vi "未命名 2.vi"() -> ()   [LabVIEW 2010]
panel:
  out "bStop":bool
  out "bRece":bool
  out "bSend":bool
  out "tmp":string
  out "第几个":i32
  out "第几组":i32
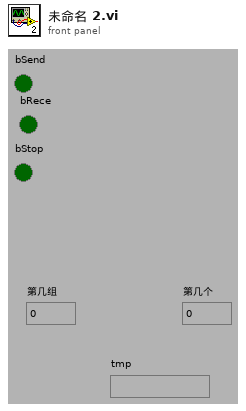
[diagram p1: front panel]
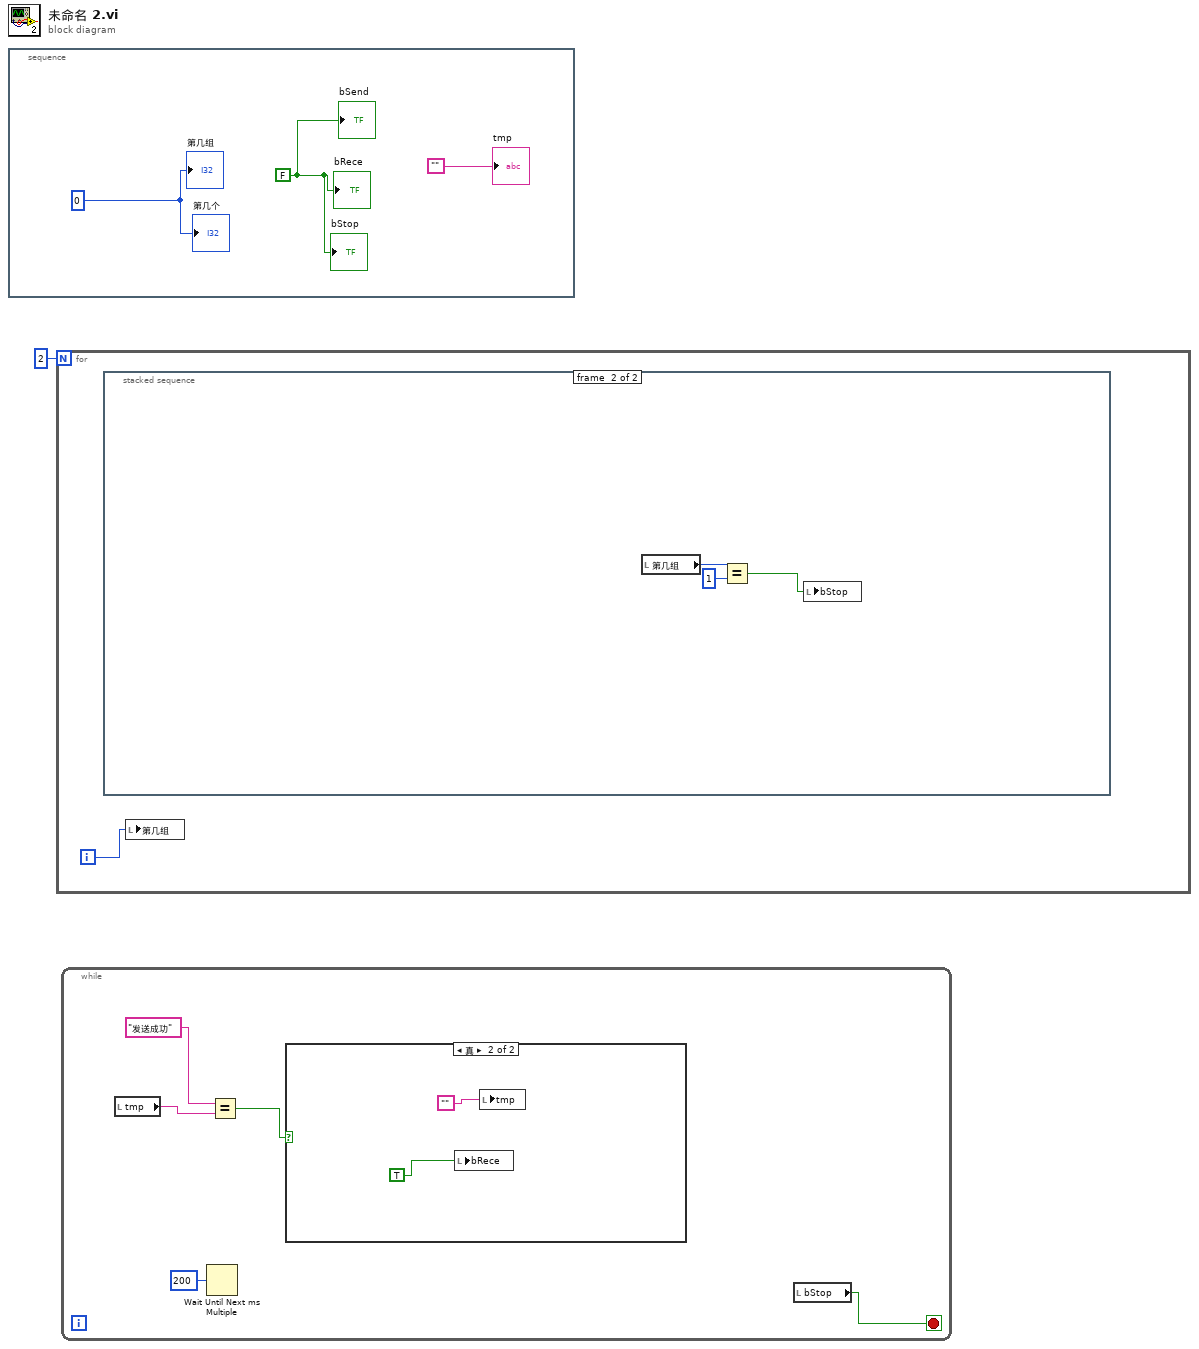
[diagram p0: block diagram]
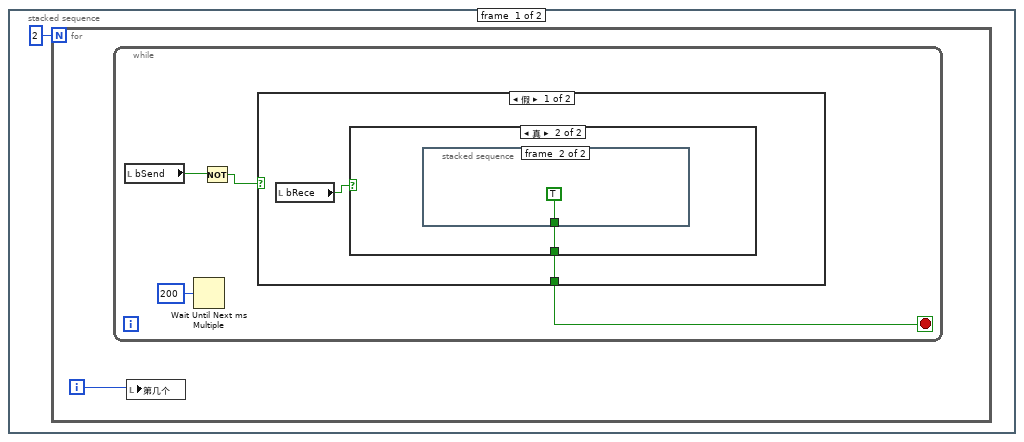
[diagram p2: hidden frame]
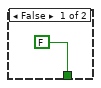
[diagram p3: hidden frame]
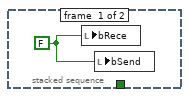
[diagram p4: hidden frame]
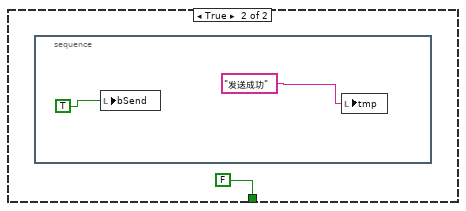
[diagram p5: hidden frame]
diagram:
  n1 = stacked-sequence {
    frame #0 {
      w2 = FALSE
      w4 = 0
      "第几组" <- w4
      "第几个" <- w4
      "tmp" <- ""
      "bSend" <- w2
      "bRece" <- w2
      "bStop" <- w2
    }
  }
  n2 = for {
    N: 2 -> [_]
    i -> [w5]
    n3 = stacked-sequence {
      frame #0 {
        n4 = for {
          N: 2 -> [_]
          i -> [w7]
          n5 = while {
            stop <- w9 stop-if-true
            n6 = local read "bSend"() -> (w11:bool)
            n7 = Wait Until Next ms Multiple(millisecond multiple=u32 200 ("毫秒倍数")) -> ()  [unwired: 1 out]
            n8 = Not(x=w11) -> (.not. x?=w10:bool)
            n9 = case shown="假" w10 {
              tunnel: [w12 FALSE] -> w9
              frame False {
                n10 = local read "bRece"() -> (w13:bool)
                n11 = case shown="真" w13 {
                  tunnel: [FALSE w15] -> w12
                  frame False {
                  }
                  frame True {
                    n12 = stacked-sequence {
                      tunnel: [_ TRUE] -> w15
                      frame #0 {
                        w16 = FALSE
                        n13 = local write "bRece"(w16) -> ()
                        n14 = local write "bSend"(w16) -> ()
                      }
                      frame #1 {
                      }
                    }
                  }
                }
              }
              frame True {
                n15 = stacked-sequence {
                  frame #0 {
                    n16 = local write "bSend"(TRUE) -> ()
                    n17 = local write "tmp"("发送成功" ("tmp 2")) -> ()
                  }
                }
              }
            }
          }
          n18 = local write "第几个"(w7) -> ()
        }
      }
      frame #1 {
        n19 = local read "第几组"() -> (w23:i32)
        n20 = Equal?(x=1 ("y"), y=w23) -> (x = y?=w21:bool)
        n21 = local write "bStop"(w21) -> ()
      }
    }
    n22 = local write "第几组"(w5) -> ()
  }
  n23 = while {
    stop <- w25 stop-if-true
    n24 = local read "tmp"() -> (w27:string)
    n25 = Wait Until Next ms Multiple(millisecond multiple=u32 200 ("毫秒倍数")) -> ()  [unwired: 1 out]
    n26 = Equal?(x="发送成功" ("tmp 2"), y=w27) -> (x = y?=w26:bool)
    n27 = case shown="真" w26 {
      frame False {
      }
      frame True {
        n28 = local write "bRece"(TRUE) -> ()
        n29 = local write "tmp"("") -> ()
      }
    }
    n30 = local read "bStop"() -> (w25:bool)
  }
